vi "dll_path.vi"() -> (2 "dll":path=path "C:/code/LabVIEW-MIDI-XPLAT/dist/TomMIDIllan_64.dll")   [LabVIEW 2020, in "LabVIEW-MIDI-XPLAT.lvclass"]
uses:
  LabVIEW-MIDI-XPLAT.lvclass
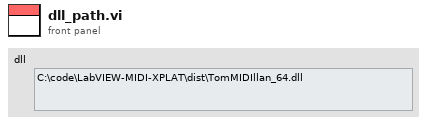
[diagram p1: front panel]
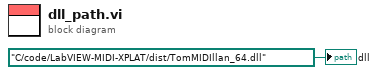
[diagram p0: block diagram]
diagram:
  "dll" <- path "C:/code/LabVIEW-MIDI-XPLAT/dist/TomMIDIllan_64.dll" ("dll")
